vi "4_0_Signal operation in Time domain.vi"() -> ()   [LabVIEW 2009]
doc: "SIGNAL OPERATION allows users to generate and analyse signals and mathematical functions that operate on them."
uses:
  Instance          30 43Saved   4_0_Signal operation in Time domain .vi
  Instance          22 43Saved   4_0_Signal operation in Time domain .vi
  Instance          21 43Saved   4_0_Signal operation in Time domain .vi
  <vilib>/Analysis/2dsp.llb/1D Convolution (DBL).vi
  <vilib>/Analysis/2dsp.llb/1D Cross Correlation (DBL).vi
  <vilib>/Analysis/2dsp.llb/1D Auto Correlation (DBL).vi
  Instance          20 43Saved   4_0_Signal operation in Time domain .vi
  Instance          17 43Saved   4_0_Signal operation in Time domain .vi
  Instance          16 43Saved   4_0_Signal operation in Time domain .vi
  Instance          18 43Saved   4_0_Signal operation in Time domain .vi
  Instance          19 43Saved   4_0_Signal operation in Time domain .vi
  Instance          13 43Saved   4_0_Signal operation in Time domain .vi
  Instance          14 43Saved   4_0_Signal operation in Time domain .vi
  Instance          15 43Saved   4_0_Signal operation in Time domain .vi
  <vilib>/Analysis/NI_AALBase.lvlib
  <vilib>/Analysis/NI_AALPro.lvlib
panel:
  out "?":string="MULTIPLICATION\nPRESS \"SUPERIMPOSE\" TO SUPERIMPOSE SIGNALS"
  out "?":bool
  out "?":string="Time"
  out "?":string="Time"
  in  "?":bool
  in  "?":bool
  out "?":string="Sine wave.    Digitalized frequency = analog freq/sampling rate"
  out "?":string="Sine wave.    Digitalized frequency = analog freq/sampling rate"
  in  "alpha":dbl=0.95
  in  "c":dbl=1.0
  in  "Freq in cycles":dbl=1.0
  in  "Samp freq Fs":dbl=1000.0
  in  "Frequency Type":enum16{"Cycles", "Hz"}(ring)=enum."Hz"
  in  "Samp freq Fs":dbl=100.0
  in  "Freq in cycles":dbl=2.0
  in  "Frequency Type":enum16{"Cycles", "Hz"}(ring)=enum."Hz"
  in  "?":bool=TRUE
  out "OUTPUT ARRAY":dbl[](array[numeric])=[0.0, 0.036907341363112925, 0.11919898848967402, 0.1782102202687055, 0.14617624806978086, 1.640005609034487e-17, -0.2163781830748172, -0.40494016974649644, -0.45817497100356813, -0.3149510878717969, -6.238952084931405e-17, 0.3746684206317084, 0.6510429858044683, 0.6932903632838676, 0.452896320799659, 1.288077127857828e-16, -0.49628350270878235, -0.8334171783286888, -0.8605416643679448, -0.5465089063334351, -2.0189673055202066e-16, 0.5693188977302334, 0.9342106906791706, 0.9435571515973541, 0.5866253923638434, 2.653584817158272e-16, -0.5866253923638429, -0.9435571515973541, -0.934210690679171, -0.5693188977302339, -3.028450958280311e-16, 0.546508906333435, 0.860541664367945, 0.8334171783286893, 0.49628350270878313, 3.005513298334935e-16, -0.45289632079965925, -0.6932903632838684, -0.6510429858044695, -0.37466842063170946, -2.495580833972569e-16, 0.3149510878717977, 0.45817497100356985, 0.40494016974649855, 0.21637818307481868, 1.47600504813105e-16, -0.14617624806978222, -0.17821022026870806, -0.11919898848967671, -0.036907341363114674, -1.6077664410013713e-30, -0.03690734136311106, -0.11919898848967093, -0.17821022026870242, -0.146176248069779, -1.8040061699379165e-16, 0.2163781830748151, 0.40494016974649316, 0.45817497100356497, 0.3149510878717951, 3.743371250958822e-16, -0.3746684206317062, -0.6510429858044651, -0.6932903632838647, -0.45289632079965764, -5.5816675540505695e-16, 0.49628350270878047, 0.8334171783286862, 0.8605416643679429, 0.5465089063334344, 7.066385569320712e-16, -0.5693188977302323, -0.9342106906791695, -0.9435571515973538, -0.5866253923638437, -7.960754451474816e-16, 0.5866253923638426, 0.9435571515973542, 0.9342106906791715, 0.5693188977302346, 8.075869222080832e-16, -0.5465089063334346, -0.8605416643679449, -0.8334171783286893, -0.4962835027087831, -7.299103724527691e-16, 0.45289632079965814, 0.6932903632838667, 0.6510429858044675, 0.3746684206317082, 5.615056876438249e-16, -0.3149510878717952, -0.45817497100356575, -0.40494016974649394, -0.21637818307481566, -3.1160106571654887e-16, 0.14617624806977822, 0.17821022026870112, 0.11919898848966928, 0.03690734136310978]
  in  "Time Delay":dbl(slide) scale=0.0..1.0
  in  "?":T1(ring)=enum."BOTH SIGNALS"
  in  "?":bool
  in  "?":bool
  in  "stop":bool
  in  "?":T2(ring)=enum."MULTIPLICATION"
  in  "Delta t":dbl=0.1 format="%0.2f"
  in  "Width":i32=10
  in  "Wave Table":dbl[](array[numeric])=[1.0, 2.0, 3.0, 4.0]
  in  "Delta t":dbl=0.1 format="%0.2f"
  in  "Width":i32=1
  in  "Wave Table":dbl[](array[numeric])=[1.0, 2.0, 2.0, 3.0]
  in  "Delay":i32(knob)=15 scale=0.0..100.0
  in  "Signal 2 Pattern":T3(ring)
  in  "Delay":i32(knob) scale=0.0..100.0
  in  "Start":dbl format="%0.2f"
  in  "End":dbl=1.0 format="%0.2f"
  in  "Start":dbl format="%0.2f"
  in  "End":dbl=1.0 format="%0.2f"
  in  "Duty cycle (%)":dbl(knob)=50.0 step=1.0 scale=0.0..100.0
  in  "Duty cycle (%)":dbl=57.0 step=1.0
  in  "Phase in":dbl(knob) scale=0.0..180.0
  in  "Frequency in Hz":dbl(knob)=100.0 scale=0.0..5000.0 scale format="%#_6p"
  in  "Amplitude":dbl=1.0
  in  "Reset phase":bool=TRUE
  in  "Samples":i32=128
  in  "Phase in":dbl(knob) scale=0.0..180.0
  in  "Frequency in Hz":dbl(knob)=1.0 scale=0.0..5000.0 scale format="%#_6p"
  in  "Amplitude":dbl=1.0
  in  "Reset phase":bool=TRUE
  in  "Samples":i32=100
  in  "Signal 1 Pattern":T4(ring)
  out "Signal Operation (x,y)":dynamicdata(graph)=[{"t0"=timestamp(0 s since 1904-01-01), "dt"=1.0, "Y"=[0.0, 0.036907341363112925, 0.11919898848967402, 0.1782102202687055, 0.14617624806978086, 1.640005609034487e-17, -0.2163781830748172, -0.40494016974649644, -0.45817497100356813, -0.3149510878717969, -6.238952084931405e-17, 0.3746684206317084, 0.6510429858044683, 0.6932903632838676, 0.452896320799659, 1.288077127857828e-16, -0.49628350270878235, -0.8334171783286888, -0.8605416643679448, -0.5465089063334351, -2.0189673055202066e-16, 0.5693188977302334, 0.9342106906791706, 0.9435571515973541, 0.5866253923638434, 2.653584817158272e-16, -0.5866253923638429, -0.9435571515973541, -0.934210690679171, -0.5693188977302339, -3.028450958280311e-16, 0.546508906333435, 0.860541664367945, 0.8334171783286893, 0.49628350270878313, 3.005513298334935e-16, -0.45289632079965925, -0.6932903632838684, -0.6510429858044695, -0.37466842063170946, -2.495580833972569e-16, 0.3149510878717977, 0.45817497100356985, 0.40494016974649855, 0.21637818307481868, 1.47600504813105e-16, -0.14617624806978222, -0.17821022026870806, -0.11919898848967671, -0.036907341363114674, -1.6077664410013713e-30, -0.03690734136311106, -0.11919898848967093, -0.17821022026870242, -0.146176248069779, -1.8040061699379165e-16, 0.2163781830748151, 0.40494016974649316, 0.45817497100356497, 0.3149510878717951, 3.743371250958822e-16, -0.3746684206317062, -0.6510429858044651, -0.6932903632838647, -0.45289632079965764, -5.5816675540505695e-16, 0.49628350270878047, 0.8334171783286862, 0.8605416643679429, 0.5465089063334344, 7.066385569320712e-16, -0.5693188977302323, -0.9342106906791695, -0.9435571515973538, -0.5866253923638437, -7.960754451474816e-16, 0.5866253923638426, 0.9435571515973542, 0.9342106906791715, 0.5693188977302346, 8.075869222080832e-16, -0.5465089063334346, -0.8605416643679449, -0.8334171783286893, -0.4962835027087831, -7.299103724527691e-16, 0.45289632079965814, 0.6932903632838667, 0.6510429858044675, 0.3746684206317082, 5.615056876438249e-16, -0.3149510878717952, -0.45817497100356575, -0.40494016974649394, -0.21637818307481566, -3.1160106571654887e-16, 0.14617624806977822, 0.17821022026870112, 0.11919898848966928, 0.03690734136310978]}]
  out "Sequence y[n]":cluster{dbl, dbl, "bernoulli noise":dbl[]}(graph)={0.0, 0.001, "bernoulli noise"=[0.0, 0.5877852522924731, 0.9510565162951535, 0.9510565162951535, 0.5877852522924731, 5.307169634316544e-17, -0.587785252292473, -0.9510565162951535, -0.9510565162951536, -0.5877852522924732, -1.0614339268633088e-16, 0.587785252292473, 0.9510565162951535, 0.9510565162951536, 0.5877852522924732, 1.5921508902949633e-16, -0.587785252292473, -0.9510565162951535, -0.9510565162951536, -0.5877852522924732, -2.1228678537266177e-16, 0.5877852522924729, 0.9510565162951535, 0.9510565162951536, 0.5877852522924734, 2.653584817158272e-16, -0.5877852522924729, -0.9510565162951535, -0.9510565162951536, -0.5877852522924734, -3.1843017805899265e-16, 0.5877852522924729, 0.9510565162951534, 0.9510565162951536, 0.5877852522924735, 3.715018744021581e-16, -0.5877852522924728, -0.9510565162951534, -0.9510565162951536, -0.5877852522924735, -4.2457357074532354e-16, 0.5877852522924728, 0.9510565162951534, 0.9510565162951538, 0.5877852522924735, 4.77645267088489e-16, -0.5877852522924727, -0.9510565162951534, -0.9510565162951538, -0.5877852522924736, -5.307169634316544e-16, 0.5877852522924727, 0.9510565162951534, 0.9510565162951538, 0.5877852522924736, 5.837886597748199e-16, -0.5877852522924727, -0.9510565162951534, -0.9510565162951538, -0.5877852522924736, -6.368603561179853e-16, 0.5877852522924726, 0.9510565162951534, 0.9510565162951538, 0.5877852522924737, 6.899320524611507e-16, -0.5877852522924726, -0.9510565162951533, -0.9510565162951538, -0.5877852522924737, -7.430037488043162e-16, 0.5877852522924725, 0.9510565162951533, 0.9510565162951539, 0.5877852522924738, 7.960754451474816e-16, -0.5877852522924725, -0.9510565162951533, -0.9510565162951539, -0.5877852522924738, -8.491471414906471e-16, 0.5877852522924725, 0.9510565162951533, 0.9510565162951539, 0.5877852522924738, 9.022188378338125e-16, -0.5877852522924724, -0.9510565162951533, -0.9510565162951539, -0.5877852522924739, -9.55290534176978e-16, 0.5877852522924724, 0.9510565162951533, 0.9510565162951539, 0.5877852522924739, 1.0083622305201434e-15, -0.5877852522924724, -0.9510565162951533, -0.9510565162951539, -0.587785252292474, -1.0614339268633088e-15, 0.5877852522924722, 0.9510565162951532, 0.9510565162951539, 0.587785252292474, 1.1145056232064743e-15, -0.5877852522924722, -0.9510565162951532, -0.951056516295154, -0.587785252292474, -1.1675773195496397e-15, 0.5877852522924721, 0.9510565162951532, 0.951056516295154, 0.5877852522924741, 1.2206490158928052e-15, -0.5877852522924721, -0.9510565162951532, -0.951056516295154, -0.5877852522924741, -1.2737207122359706e-15, 0.5877852522924721, 0.9510565162951532, 0.951056516295154, 0.5877852522924742, 1.326792408579136e-15, -0.587785252292472, -0.9510565162951532]}
  out "Sequence x[n]":cluster{dbl, dbl, "Waveform Graph":dbl[]}(graph)={0.0, 0.01, "Waveform Graph"=[0.0, 0.06279051952931337, 0.12533323356430426, 0.18738131458572463, 0.2486898871648548, 0.3090169943749474, 0.368124552684678, 0.42577929156507266, 0.4817536741017153, 0.5358267949789967, 0.5877852522924732, 0.6374239897486899, 0.6845471059286888, 0.7289686274214117, 0.7705132427757894, 0.8090169943749476, 0.8443279255020152, 0.8763066800438637, 0.9048270524660196, 0.9297764858882515, 0.9510565162951535, 0.9685831611286311, 0.9822872507286886, 0.9921147013144778, 0.9980267284282716, 1.0, 0.9980267284282716, 0.9921147013144779, 0.9822872507286888, 0.9685831611286313, 0.9510565162951539, 0.9297764858882518, 0.90482705246602, 0.8763066800438643, 0.8443279255020159, 0.8090169943749483, 0.7705132427757903, 0.7289686274214127, 0.6845471059286901, 0.6374239897486912, 0.5877852522924748, 0.5358267949789984, 0.4817536741017172, 0.42577929156507477, 0.3681245526846802, 0.30901699437494984, 0.24868988716485732, 0.18738131458572732, 0.12533323356430706, 0.0627905195293163, 3.0294235002503722e-15, -0.06279051952931025, -0.12533323356430104, -0.18738131458572135, -0.24868988716485146, -0.30901699437494407, -0.3681245526846746, -0.4257792915650693, -0.48175367410171194, -0.5358267949789933, -0.5877852522924699, -0.6374239897486865, -0.6845471059286856, -0.7289686274214086, -0.7705132427757864, -0.8090169943749448, -0.8443279255020126, -0.8763066800438613, -0.9048270524660175, -0.9297764858882496, -0.951056516295152, -0.9685831611286299, -0.9822872507286877, -0.9921147013144772, -0.9980267284282713, -1.0, -0.9980267284282718, -0.9921147013144782, -0.9822872507286892, -0.9685831611286317, -0.9510565162951542, -0.929776485888252, -0.90482705246602, -0.876306680043864, -0.8443279255020153, -0.8090169943749475, -0.770513242775789, -0.728968627421411, -0.6845471059286878, -0.6374239897486885, -0.5877852522924716, -0.5358267949789947, -0.48175367410171294, -0.4257792915650699, -0.36812455268467476, -0.30901699437494373, -0.24868988716485066, -0.18738131458572005, -0.12533323356429923, -0.06279051952930793]}
  # "Program Developed by Indranil Sinharoy"
  # "Message Box"
  # "Signal/Sequence x(n)"
  # "Real Exponential"
  # "Impulse/Pulse/Sinc\n/Step"
  # "Pulse"
  # "Sinc"
  # "Ramp char."
  # "Square Wave char."
  # "Arbitrary Waveform (Point by Point)"
  # "SIGNAL OPERATION"
  # "Signal/Sequence y(n)"
  # "Pulse"
  # "Sinc"
  # "Square Wave char."
  # "Impulse/Pulse/Sinc\n/Step"
  # "Ramp char."
  # "Arbitrary Waveform (Point by Point)"
  # "y[n]"
  # "x[n]"
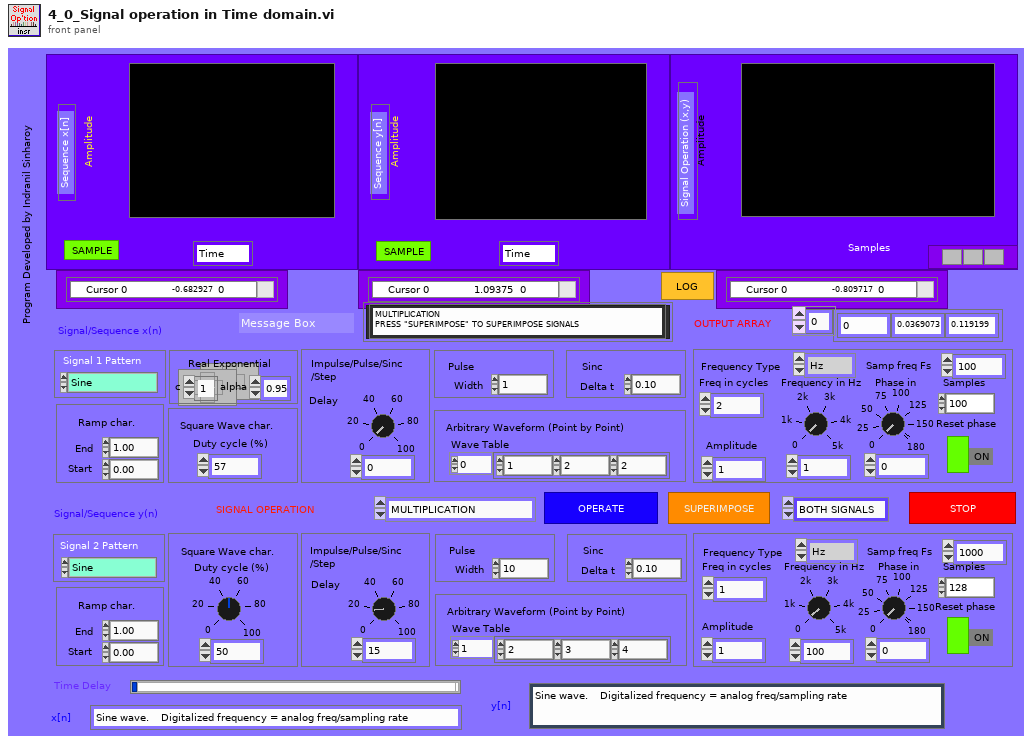
[diagram p1: front panel]
types:
  T1 = enum16{"NO SIGNAL", "SIGNAL x[n]", "SIGNAL y[n]", "BOTH SIGNALS"}
  T2 = enum16{"CONVOLUTION", "ADDITION", "MULTIPLICATION", "CROSS CORRELATION", "AUTO CORRELATION", "BACKWARD DIFFERENCE", "ACCUMULATOR FUNCTION"}
  T3 = enum16{"Sine", "Square", "Ramp", "Triangular", "Sawtooth", "Pulse wave", "Impulse", "Step", "Sinc Pattern", "Arbitrary wave", "Unif. white noise", "Gaussian white noise", "Periodic rand noise", "Gamma noise", "Poisson noise", "Binomial noise", "Bernoulli noise"}
  T4 = enum16{"Sine", "Square", "Ramp", "Triangular", "Sawtooth", "Pulse wave", "Impulse", "Step", "Sinc Pattern", "Arbitrary wave", "Real Exponential", "Chirp Pattern"}
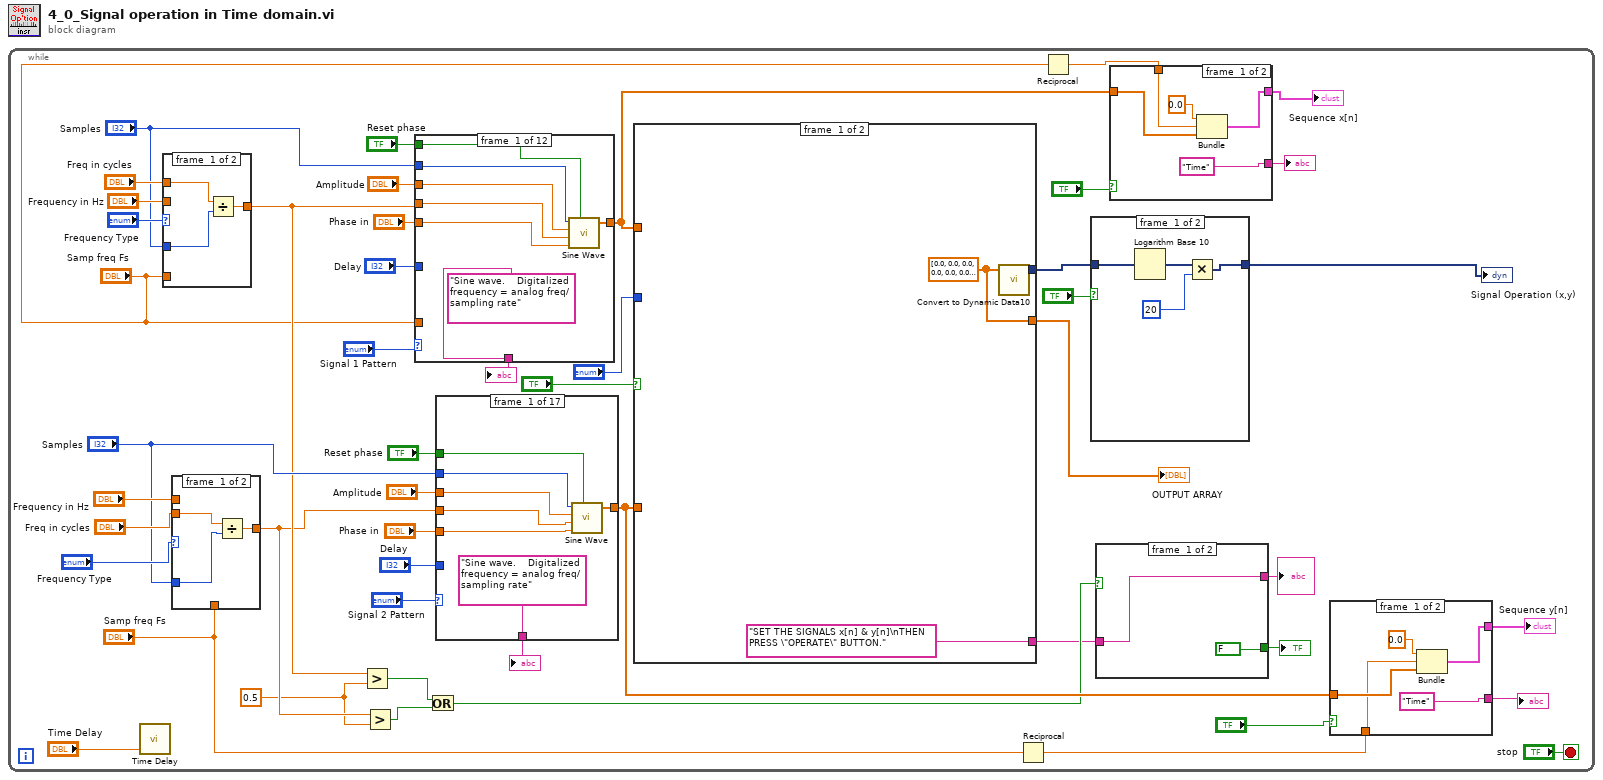
[diagram p0: block diagram]
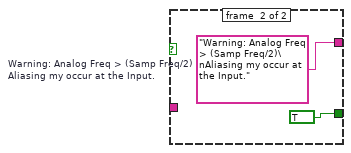
[diagram p2: hidden frame]
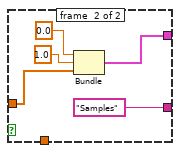
[diagram p3: hidden frame]
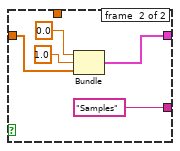
[diagram p4: hidden frame]
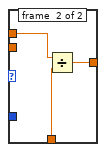
[diagram p5: hidden frame]
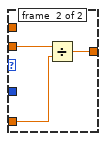
[diagram p6: hidden frame]
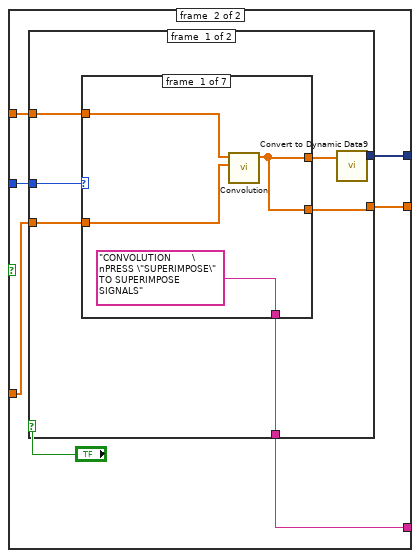
[diagram p8: hidden frame]
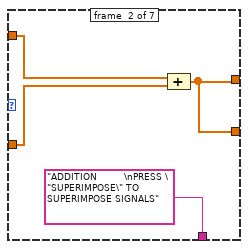
[diagram p9: hidden frame]
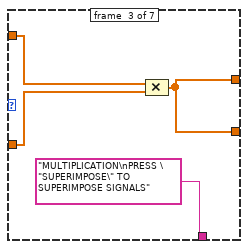
[diagram p10: hidden frame]
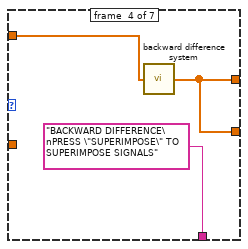
[diagram p11: hidden frame]
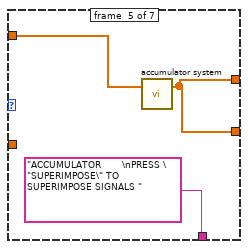
[diagram p12: hidden frame]
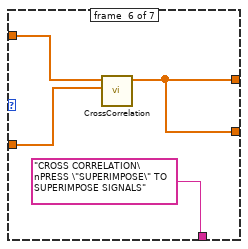
[diagram p13: hidden frame]
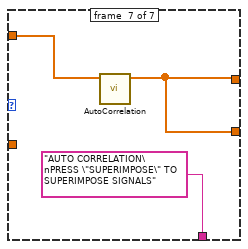
[diagram p14: hidden frame]
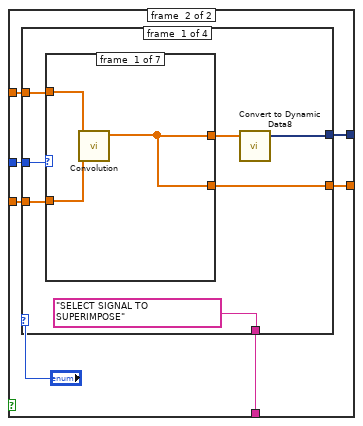
[diagram p15: hidden frame]
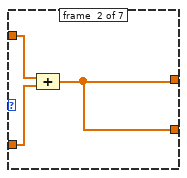
[diagram p16: hidden frame]
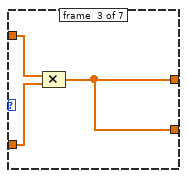
[diagram p17: hidden frame]
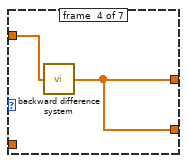
[diagram p18: hidden frame]
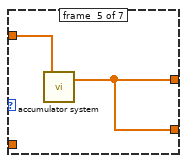
[diagram p19: hidden frame]
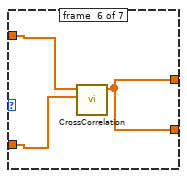
[diagram p20: hidden frame]
diagram:
  n1 = while {
    stop <- "stop" stop-if-true
    w6 = 0.5
    n2 = call "Time Delay"("Delay Time (s)"="Time Delay") -> ()  [unwired: 10 in, 1 out]
    n3 = case shown="\"Cycles\", Default" "Frequency Type" {
      tunnel: "Frequency in Hz" -> [_ w85]
      tunnel: "Freq in cycles" -> [w81 _]
      tunnel: "Samp freq Fs" -> [_ w84]
      tunnel: [w82 w83] -> w9
      tunnel: "Samples" -> [w80 _]
      frame #0 {
        n4 = Divide(x=w81, y=w80) -> (x/y=w82:dbl)
      }
      frame #1 {
        n5 = Divide(x=w85, y=w84) -> (x/y=w83:dbl)
      }
    }
    n6 = case shown="\"Cycles\", Default" "Frequency Type" {
      tunnel: [w76 w79] -> w7
      tunnel: "Frequency in Hz" -> [_ w78]
      tunnel: "Freq in cycles" -> [w75 _]
      tunnel: "Samp freq Fs" -> [_ w77]
      tunnel: "Samples" -> [w74 _]
      frame #0 {
        n7 = Divide(x=w75, y=w74) -> (x/y=w76:dbl)
      }
      frame #1 {
        n8 = Divide(x=w78, y=w77) -> (x/y=w79:dbl)
      }
    }
    n9 = Greater?(x=w9, y=w6) -> (0:w11:bool)
    n10 = Greater?(x=w7, y=w6) -> (0:w10:bool)
    n11 = case shown="\"Chirp Pattern\"" "Signal 1 Pattern" {
      tunnel: "Samples" -> [w377 w384 w390 w396 w403 w409 _ w417 w423 w427 w432 w439]
      tunnel: "Reset phase" -> [w376 w385 _ w397 w404 _ _ _ _ _ _ _]
      tunnel: "Amplitude" -> [w375 w383 _ w395 w402 w408 _ w416 w422 _ _ w438]
      tunnel: w9 -> [w374 w382 _ w394 w401 _ _ _ _ _ _ w434]
      tunnel: "Phase in" -> [w373 w381 _ w393 w400 _ _ _ _ _ _ _]
      tunnel: [w372 w380 w389 w392 w399 w407 "Wave Table" w414 w420 w425 w429 w440] -> w36
      tunnel: "Delay" -> [_ _ _ _ _ w406 _ w415 w421 w426 _ w437]
      tunnel: ["Sine wave.    Digitalized frequency = analog freq/sampling rate" "Square wave.    Digitalized frequency = analog freq/sampling rate" " Ramp.    Digitalized frequency = analog freq/sampling rate" "Triangular wave.    Digitalized frequency = analog freq/sampling rate" "Sawtooth wave.    Digitalized frequency = analog freq/sampling rate" "Impulse Function. Vary the delay to generate impulse at delayed instant." "Create arbitrary sequence by specifying values in the wave table" "Pulse. Vary the delay to generate Pulse at delayed instant." "Sinc pattern. Vary the delay to generate sinc at delayed instant." "Step function. Vary the delay to generate step at delayed instant." w428 "Chirp pattern. Vary delay knob to set f1 & freq knob to set f2."] -> w8
      tunnel: "Samp freq Fs" -> [_ _ _ _ _ _ _ _ _ _ _ w436]
      frame #0 {
        n12 = call <vilib>:"Sine Wave.vi"("samples"=w377, "amplitude"=w375, "frequency"=w374, "phase in"=w373, "reset phase"=w376) -> ("sine wave"=w372:dbl[])  [unwired: 2 out]
      }
      frame #1 {
        n13 = call <vilib>:"Square Wave.vi"("samples"=w384, "reset phase"=w385, "amplitude"=w383, "frequency"=w382, "duty cycle (%)"="Duty cycle (%)", "phase in"=w381) -> ("square wave"=w380:dbl[])  [unwired: 2 out]
      }
      frame #2 {
        n14 = call <vilib>:"Ramp Pattern.vi"("start"="Start", "end"="End", "samples"=w390) -> ("Ramp Pattern"=w389:dbl[])  [unwired: 7 in, 1 out]
      }
      frame #3 {
        n15 = call <vilib>:"Triangle Wave.vi"("samples"=w396, "amplitude"=w395, "frequency"=w394, "phase in"=w393, "reset phase"=w397) -> ("triangle wave"=w392:dbl[])  [unwired: 2 out]
      }
      frame #4 {
        n16 = call <vilib>:"Sawtooth Wave.vi"("samples"=w403, "amplitude"=w402, "frequency"=w401, "phase in"=w400, "reset phase"=w404) -> ("sawtooth wave"=w399:dbl[])  [unwired: 2 out]
      }
      frame #5 {
        n17 = call <vilib>:"Impulse Pattern.vi"("delay"=w406, "amplitude"=w408, "samples"=w409) -> ("Impulse Pattern"=w407:dbl[])  [unwired: 1 out]
      }
      frame #6 {
      }
      frame #7 {
        n18 = call <vilib>:"Pulse Pattern.vi"("width"="Width", "delay"=w415, "amplitude"=w416, "samples"=w417) -> ("Pulse Pattern"=w414:dbl[])  [unwired: 1 out]
      }
      frame #8 {
        n19 = call <vilib>:"Sinc Pattern.vi"("delta t"="Delta t", "delay"=w421, "amplitude"=w422, "samples"=w423) -> ("Sinc Pattern"=w420:dbl[])  [unwired: 1 out]
      }
      frame #9 {
        n20 = call "stepinput_numarray.vi"("Step Delay"=w426, "Samples"=w427) -> ("OUTPUT ARRAY"=w425:dbl[])
      }
      frame #10 {
        w428 = "Real exponential sequence  x[n] = C*alpha^n"  # Real exponential sequence  x[n] = C*alpha^n
        n21 = call "C alpha to the power n.vi"("alpha"="alpha", "c"="c", "n"=w432) -> ("Waveform Graph"=w429:dbl[])
      }
      frame #11 {
        n22 = Divide(x=w437, y=w436) -> (x/y=w435:dbl)
        n23 = call <vilib>:"Chirp Pattern.vi"("f2"=w434, "f1"=w435, "amplitude"=w438, "samples"=w439) -> ("Chirp Pattern"=w440:dbl[])  [unwired: 1 out]
      }
    }
    "?" <- w8
    n24 = Or(x=w11, y=w10) -> (x .or. y?=w5:bool)
    n25 = case shown="\"Sinc Pattern\"" "Signal 2 Pattern" {
      tunnel: "Reset phase" -> [w284 w287 _ w304 w310 _ _ _ _ _ _ _ _ _ _ _ _]
      tunnel: "Samples" -> [w283 w288 w297 w303 w309 w317 w320 w328 _ w334 w339 w343 w348 w353 w358 w364 w369]
      tunnel: "Amplitude" -> [w282 w289 _ w302 w308 w316 w321 w327 _ _ w338 _ w347 _ _ _ _]
      tunnel: "Phase in" -> [w281 w290 _ w301 w307 _ _ _ _ _ _ _ _ _ _ _ _]
      tunnel: [w280 w291 w296 w300 w311 w314 w319 w325 "Wave Table" w333 w337 w344 w349 w354 w359 w365 w370] -> w15
      tunnel: "Delay" -> [_ _ _ _ _ w315 w322 w326 _ w332 _ _ _ _ _ _ _]
      tunnel: w7 -> [w279 w286 _ w299 w306 _ _ _ _ _ _ _ _ _ _ _ _]
      tunnel: ["Sine wave.    Digitalized frequency = analog freq/sampling rate" "Square wave.    Digitalized frequency = analog freq/sampling rate" " Ramp.    Digitalized frequency = analog freq/sampling rate" "Triangular wave.    Digitalized frequency = analog freq/sampling rate" "Sawtooth wave.    Digitalized frequency = analog freq/sampling rate" "Pulse. Vary the delay to generate Pulse at delayed instant." "Impulse Function. Vary the delay to generate impulse at delayed instant." "Sinc pattern. Vary the delay to generate sinc at delayed instant." "Create arbitrary sequence by specifying values in the wave table" "Step function. Vary the delay to generate step at delayed instant." "Uniform White Noise. Seed has been set to -1. The amplitude & no. of samples can be varied." "Gaussian White Noise. Seed has been set to -1, standard deviation to 1. The no. of samples can be varied." "Periodic Random Noise. Seed has been set to -1. The amplitude & no. of samples can be varied." "Gamma Noise. Seed has been set to -1, order to 1. The no. of samples can be varied." "Poisson Noise. Seed has been set to -1, mean to 1. The no. of samples can be varied." "Binomial Noise. Seed has been set to -1, trials to 1 and trial probability to 0.5 . The no. of samples can be varied." "Bernoulli Noise. Seed has been set to -1 and ones probability to 0.5 . The no. of samples can be varied."] -> w23
      frame #0 {
        n26 = call <vilib>:"Sine Wave.vi"("samples"=w283, "amplitude"=w282, "frequency"=w279, "phase in"=w281, "reset phase"=w284) -> ("sine wave"=w280:dbl[])  [unwired: 2 out]
      }
      frame #1 {
        n27 = call <vilib>:"Square Wave.vi"("samples"=w288, "reset phase"=w287, "amplitude"=w289, "frequency"=w286, "duty cycle (%)"="Duty cycle (%)", "phase in"=w290) -> ("square wave"=w291:dbl[])  [unwired: 2 out]
      }
      frame #2 {
        n28 = call <vilib>:"Ramp Pattern.vi"("start"="Start", "end"="End", "samples"=w297) -> ("Ramp Pattern"=w296:dbl[])  [unwired: 7 in, 1 out]
      }
      frame #3 {
        n29 = call <vilib>:"Triangle Wave.vi"("samples"=w303, "amplitude"=w302, "frequency"=w299, "phase in"=w301, "reset phase"=w304) -> ("triangle wave"=w300:dbl[])  [unwired: 2 out]
      }
      frame #4 {
        n30 = call <vilib>:"Sawtooth Wave.vi"("samples"=w309, "amplitude"=w308, "frequency"=w306, "phase in"=w307, "reset phase"=w310) -> ("sawtooth wave"=w311:dbl[])  [unwired: 2 out]
      }
      frame #5 {
        n31 = call <vilib>:"Pulse Pattern.vi"("width"="Width", "delay"=w315, "amplitude"=w316, "samples"=w317) -> ("Pulse Pattern"=w314:dbl[])  [unwired: 1 out]
      }
      frame #6 {
        n32 = call <vilib>:"Impulse Pattern.vi"("delay"=w322, "amplitude"=w321, "samples"=w320) -> ("Impulse Pattern"=w319:dbl[])  [unwired: 1 out]
      }
      frame #7 {
        n33 = call <vilib>:"Sinc Pattern.vi"("delta t"="Delta t", "delay"=w326, "amplitude"=w327, "samples"=w328) -> ("Sinc Pattern"=w325:dbl[])  [unwired: 1 out]
      }
      frame #8 {
      }
      frame #9 {
        n34 = call "stepinput_numarray.vi"("Step Delay"=w332, "Samples"=w334) -> ("OUTPUT ARRAY"=w333:dbl[])
      }
      frame #10 {
        n35 = call <vilib>:"Uniform White Noise (obs 90).vi"("seed"=-1, "amplitude"=w338, "samples"=w339) -> ("uniform white noise"=w337:dbl[])  [unwired: 1 out]
      }
      frame #11 {
        n36 = call <vilib>:"Gaussian White Noise (obs 90).vi"("seed"=-1, "standard deviation"=1.0000000000000002, "samples"=w343) -> ("Gaussian noise pattern"=w344:dbl[])  [unwired: 1 out]
      }
      frame #12 {
        n37 = call <vilib>:"Periodic Random Noise.vi"("seed"=-1, "spectral amplitude"=w347, "samples"=w348) -> ("periodic random noise"=w349:dbl[])  [unwired: 1 out]
      }
      frame #13 {
        n38 = call <vilib>:"Gamma Noise (obs 90).vi"("seed"=-1, "order"=1, "samples"=w353) -> ("gamma noise"=w354:dbl[])  [unwired: 1 out]
      }
      frame #14 {
        n39 = call <vilib>:"Poisson Noise (obs 90).vi"("seed"=-1, "mean"=1.0, "samples"=w358) -> ("poisson noise"=w359:dbl[])  [unwired: 1 out]
      }
      frame #15 {
        n40 = call <vilib>:"Binomial Noise (obs 90).vi"("seed"=-1, "trial probability"=0.5, "trials"=1, "samples"=w364) -> ("binomial noise"=w365:u32[])  [unwired: 1 out]
      }
      frame #16 {
        n41 = call <vilib>:"Bernoulli Noise (obs 90).vi"("seed"=-1, "ones probability"=0.5, "samples"=w369) -> ("bernoulli noise"=w370:u8[])  [unwired: 1 out]
      }
    }
    "?" <- w23
    n42 = case shown="True" "?" {
      tunnel: "?" -> [_ w100]
      tunnel: w36 -> [_ w99]
      tunnel: w15 -> [_ w98]
      tunnel: [w93 w96] -> w33
      tunnel: ["SET THE SIGNALS x[n] & y[n]\nTHEN PRESS \"OPERATE\" BUTTON." w95] -> w4
      tunnel: [w91 w94] -> w34
      frame #0 {
        w91 = dbl[] [0.0, 0.0, 0.0, 0.0, 0.0, 0.0, 0.0, 0.0, 0.0, 0.0, 0.0, 0.0, 0.0, 0.0, 0.0, 0.0, 0.0, 0.0, 0.0, 0.0, 0.0, 0.0, 0.0, 0.0, 0.0, 0.0, 0.0, 0.0, 0.0, 0.0, 0.0, 0.0, 0.0, 0.0, 0.0, 0.0, 0.0, 0.0, 0.0, 0.0, 0.0, 0.0, 0.0, 0.0, 0.0, 0.0, 0.0, 0.0, 0.0, 0.0, 0.0, 0.0, 0.0, 0.0, 0.0, 0.0, 0.0, 0.0, 0.0, 0.0, 0.0, 0.0, 0.0, 0.0, 0.0, 0.0, 0.0, 0.0, 0.0, 0.0, 0.0, 0.0, 0.0, 0.0, 0.0, 0.0, 0.0, 0.0, 0.0, 0.0, 0.0, 0.0, 0.0, 0.0, 0.0, 0.0, 0.0, 0.0, 0.0, 0.0, 0.0, 0.0, 0.0, 0.0, 0.0, 0.0, 0.0, 0.0, 0.0, 0.0, 0.0] ("X * Y")
        n43 = call "Convert to Dynamic Data10"("Array"=w91) -> ("Dynamic Data Type"=w93:dynamicdata)  [unwired: 3 in]
      }
      frame #1 {
        n44 = case shown="True" "?" {
          tunnel: w100 -> [w105 w139]
          tunnel: w99 -> [w107 w138]
          tunnel: w98 -> [w106 w137]
          tunnel: [w103 w135] -> w96
          tunnel: [w102 w134] -> w95
          tunnel: [w101 w133] -> w94
          frame #0 {
            n45 = case shown="\"MULTIPLICATION\"" w105 {
              tunnel: w107 -> [w111 w115 w119 w122 w125 w128 w131]
              tunnel: w106 -> [w110 w114 w118 _ _ w126 _]
              tunnel: [w108 w112 w116 w120 w123 w127 w130] -> w104
              tunnel: ["CONVOLUTION       \nPRESS \"SUPERIMPOSE\" TO SUPERIMPOSE SIGNALS" "ADDITION         \nPRESS \"SUPERIMPOSE\" TO SUPERIMPOSE SIGNALS" "MULTIPLICATION\nPRESS \"SUPERIMPOSE\" TO SUPERIMPOSE SIGNALS" "BACKWARD DIFFERENCE\nPRESS \"SUPERIMPOSE\" TO SUPERIMPOSE SIGNALS" "ACCUMULATOR       \nPRESS \"SUPERIMPOSE\" TO SUPERIMPOSE SIGNALS " "CROSS CORRELATION\nPRESS \"SUPERIMPOSE\" TO SUPERIMPOSE SIGNALS" "AUTO CORRELATION\nPRESS \"SUPERIMPOSE\" TO SUPERIMPOSE SIGNALS"] -> w102
              tunnel: [w108 w112 w116 w120 w123 w127 w130] -> w101
              frame #0 {
                n46 = call-poly <vilib>:"Convolution.vi"("Y"=w110, "X"=w111) -> ("X * Y"=w108:dbl[])  [unwired: 8 in, 1 out]
              }
              frame #1 {
                n47 = Compound Arithmetic op=ADD(w115, w114) -> (w112:dbl[])
              }
              frame #2 {
                n48 = Compound Arithmetic op=MULTIPLY(w119, w118) -> (w116:dbl[])
              }
              frame #3 {
                n49 = call "backward difference system.vi"("Input sequence x[n]"=w122) -> ("B[n] = x[n] - x[n-1]"=w120:dbl[])
              }
              frame #4 {
                n50 = call "accumulator system.vi"("Sequence x[n]"=w125) -> ("Accumulated sequence A[n] = Sum(k: k ( -infinity to n) x[k]"=w123:dbl[])  [unwired: 2 out]
              }
              frame #5 {
                n51 = call-poly <vilib>:"CrossCorrelation.vi"("Y"=w126, "X"=w128) -> ("Rxy"=w127:dbl[])  [unwired: 8 in, 1 out]
              }
              frame #6 {
                n52 = call-poly <vilib>:"AutoCorrelation.vi"("X"=w131) -> ("Rxx"=w130:dbl[])  [unwired: 9 in, 1 out]
              }
            }
            n53 = call "Convert to Dynamic Data9"("Array"=w104) -> ("Dynamic Data Type"=w103:dynamicdata)  [unwired: 3 in]
          }
          frame #1 {
            n54 = case shown="\"SIGNAL x[n]\"" "?" {
              tunnel: w139 -> [w144 w174 w207 w247]
              tunnel: w138 -> [w146 w173 w209 w249]
              tunnel: w137 -> [w145 w172 w208 w248]
              tunnel: [w142 w167 w202 w240] -> w135
              tunnel: ["SELECT SIGNAL TO SUPERIMPOSE" w166 w201 w239] -> w134
              tunnel: [w140 w165 w200 w238] -> w133
              frame #0 {
                n55 = case shown="\"MULTIPLICATION\"" w144 {
                  tunnel: w146 -> [w149 w152 w155 w157 w159 w161 w163]
                  tunnel: w145 -> [w148 w151 w154 _ _ w160 _]
                  tunnel: [w147 w150 w153 w156 w158 w162 w164] -> w143
                  tunnel: [w147 w150 w153 w156 w158 w162 w164] -> w140
                  frame #0 {
                    n56 = call-poly <vilib>:"Convolution.vi"("Y"=w148, "X"=w149) -> ("X * Y"=w147:dbl[])  [unwired: 8 in, 1 out]
                  }
                  frame #1 {
                    n57 = Compound Arithmetic op=ADD(w152, w151) -> (w150:dbl[])
                  }
                  frame #2 {
                    n58 = Compound Arithmetic op=MULTIPLY(w155, w154) -> (w153:dbl[])
                  }
                  frame #3 {
                    n59 = call "backward difference system.vi"("Input sequence x[n]"=w157) -> ("B[n] = x[n] - x[n-1]"=w156:dbl[])
                  }
                  frame #4 {
                    n60 = call "accumulator system.vi"("Sequence x[n]"=w159) -> ("Accumulated sequence A[n] = Sum(k: k ( -infinity to n) x[k]"=w158:dbl[])  [unwired: 2 out]
                  }
                  frame #5 {
                    n61 = call-poly <vilib>:"CrossCorrelation.vi"("Y"=w160, "X"=w161) -> ("Rxy"=w162:dbl[])  [unwired: 8 in, 1 out]
                  }
                  frame #6 {
                    n62 = call-poly <vilib>:"AutoCorrelation.vi"("X"=w163) -> ("Rxx"=w164:dbl[])  [unwired: 9 in, 1 out]
                  }
                }
                n63 = call "Convert to Dynamic Data8"("Array"=w143) -> ("Dynamic Data Type"=w142:dynamicdata)  [unwired: 3 in]
              }
              frame #1 {
                n64 = case shown="\"MULTIPLICATION\"" w174 {
                  tunnel: w173 -> [w177 w181 w185 w189 w192 w194 w199]
                  tunnel: w172 -> [w178 w182 w186 _ _ w195 _]
                  tunnel: [w175 w179 w183 w187 w190 w196 w198] -> w169
                  tunnel: [w177 w181 w185 w189 w192 w194 w199] -> w171
                  tunnel: ["CONVOLUTION        \n" "ADDITIION        \n" "MULTIPLICATION        \n" "BACKWARD DIFFERENCE        \n" "ACCUMULATOR FUNCTION        \n" "CROSS CORRELATION" "AUTO CORRELATION"] -> w166
                  tunnel: [w175 w179 w183 w187 w190 w196 w198] -> w165
                  frame #0 {
                    n65 = call-poly <vilib>:"Convolution.vi"("Y"=w178, "X"=w177) -> ("X * Y"=w175:dbl[])  [unwired: 8 in, 1 out]
                  }
                  frame #1 {
                    n66 = Compound Arithmetic op=ADD(w181, w182) -> (w179:dbl[])
                  }
                  frame #2 {
                    n67 = Compound Arithmetic op=MULTIPLY(w185, w186) -> (w183:dbl[])
                  }
                  frame #3 {
                    n68 = call "backward difference system.vi"("Input sequence x[n]"=w189) -> ("B[n] = x[n] - x[n-1]"=w187:dbl[])
                  }
                  frame #4 {
                    n69 = call "accumulator system.vi"("Sequence x[n]"=w192) -> ("Accumulated sequence A[n] = Sum(k: k ( -infinity to n) x[k]"=w190:dbl[])  [unwired: 2 out]
                  }
                  frame #5 {
                    n70 = call-poly <vilib>:"CrossCorrelation.vi"("Y"=w195, "X"=w194) -> ("Rxy"=w196:dbl[])  [unwired: 8 in, 1 out]
                  }
                  frame #6 {
                    n71 = call-poly <vilib>:"AutoCorrelation.vi"("X"=w199) -> ("Rxx"=w198:dbl[])  [unwired: 9 in, 1 out]
                  }
                }
                n72 = call "Convert to Dynamic Data4"("Array"=w171) -> ("Dynamic Data Type"=w170:dynamicdata)  [unwired: 3 in]
                n73 = call "Convert to Dynamic Data5"("Array"=w169) -> ("Dynamic Data Type"=w168:dynamicdata)  [unwired: 3 in]
                n74 = Merge Signals(w170, w168) -> (w167:dynamicdata)
              }
              frame #2 {
                n75 = case shown="\"MULTIPLICATION\"" w207 {
                  tunnel: w209 -> [w213 w217 w221 w225 w229 w232 w237]
                  tunnel: w208 -> [w212 w216 w220 _ _ w231 w235]
                  tunnel: [w210 w214 w218 w222 w226 w233 w236] -> w203
                  tunnel: [w212 w216 w220 dbl[] [0.0, 0.0, 0.0, 0.0, 0.0, 0.0, 0.0, 0.0, 0.0, 0.0, 0.0, 0.0, 0.0, 0.0, 0.0, 0.0, 0.0, 0.0, 0.0, 0.0, 0.0, 0.0, 0.0, 0.0, 0.0, 0.0, 0.0, 0.0, 0.0, 0.0, 0.0, 0.0, 0.0, 0.0, 0.0, 0.0, 0.0, 0.0, 0.0, 0.0, 0.0, 0.0, 0.0, 0.0, 0.0, 0.0, 0.0, 0.0, 0.0, 0.0, 0.0, 0.0, 0.0, 0.0, 0.0, 0.0, 0.0, 0.0, 0.0, 0.0, 0.0, 0.0, 0.0, 0.0, 0.0, 0.0, 0.0, 0.0, 0.0, 0.0, 0.0, 0.0, 0.0, 0.0, 0.0, 0.0, 0.0, 0.0, 0.0, 0.0, 0.0, 0.0, 0.0, 0.0, 0.0, 0.0, 0.0, 0.0, 0.0, 0.0, 0.0, 0.0, 0.0, 0.0, 0.0, 0.0, 0.0, 0.0, 0.0, 0.0, 0.0] dbl[] [0.0, 0.0, 0.0, 0.0, 0.0, 0.0, 0.0, 0.0, 0.0, 0.0, 0.0, 0.0, 0.0, 0.0, 0.0, 0.0, 0.0, 0.0, 0.0, 0.0, 0.0, 0.0, 0.0, 0.0, 0.0, 0.0, 0.0, 0.0, 0.0, 0.0, 0.0, 0.0, 0.0, 0.0, 0.0, 0.0, 0.0, 0.0, 0.0, 0.0, 0.0, 0.0, 0.0, 0.0, 0.0, 0.0, 0.0, 0.0, 0.0, 0.0, 0.0, 0.0, 0.0, 0.0, 0.0, 0.0, 0.0, 0.0, 0.0, 0.0, 0.0, 0.0, 0.0, 0.0, 0.0, 0.0, 0.0, 0.0, 0.0, 0.0, 0.0, 0.0, 0.0, 0.0, 0.0, 0.0, 0.0, 0.0, 0.0, 0.0, 0.0, 0.0, 0.0, 0.0, 0.0, 0.0, 0.0, 0.0, 0.0, 0.0, 0.0, 0.0, 0.0, 0.0, 0.0, 0.0, 0.0, 0.0, 0.0, 0.0, 0.0] w231 w235] -> w204
                  tunnel: ["CONVOLUTION        \n" "ADDITION            \n" "MULTIPLICATION        \n" "BACKWARD DIFFERENCE  \n" "ACCUMULATOR         \n" "CROSS CORRELATION" "AUTO CORRELATION"] -> w201
                  tunnel: [w210 w214 w218 w222 w226 w233 w236] -> w200
                  frame #0 {
                    n76 = call-poly <vilib>:"Convolution.vi"("Y"=w212, "X"=w213) -> ("X * Y"=w210:dbl[])  [unwired: 8 in, 1 out]
                  }
                  frame #1 {
                    n77 = Compound Arithmetic op=ADD(w217, w216) -> (w214:dbl[])
                  }
                  frame #2 {
                    n78 = Compound Arithmetic op=MULTIPLY(w221, w220) -> (w218:dbl[])
                  }
                  frame #3 {
                    n79 = call "backward difference system.vi"("Input sequence x[n]"=w225) -> ("B[n] = x[n] - x[n-1]"=w222:dbl[])
                  }
                  frame #4 {
                    n80 = call "accumulator system.vi"("Sequence x[n]"=w229) -> ("Accumulated sequence A[n] = Sum(k: k ( -infinity to n) x[k]"=w226:dbl[])  [unwired: 2 out]
                  }
                  frame #5 {
                    n81 = call-poly <vilib>:"CrossCorrelation.vi"("Y"=w231, "X"=w232) -> ("Rxy"=w233:dbl[])  [unwired: 8 in, 1 out]
                  }
                  frame #6 {
                    n82 = call-poly <vilib>:"AutoCorrelation.vi"("X"=w237) -> ("Rxx"=w236:dbl[])  [unwired: 9 in, 1 out]
                  }
                }
                n83 = call "Convert to Dynamic Data6"("Array"=w203) -> ("Dynamic Data Type"=w206:dynamicdata)  [unwired: 3 in]
                n84 = call "Convert to Dynamic Data7"("Array"=w204) -> ("Dynamic Data Type"=w205:dynamicdata)  [unwired: 3 in]
                n85 = Merge Signals(w206, w205) -> (w202:dynamicdata)
              }
              frame #3 {
                n86 = case shown="\"MULTIPLICATION\"" w247 {
                  tunnel: w249 -> [w253 w257 w261 w265 w269 w271 w277]
                  tunnel: w248 -> [w252 w256 w260 _ _ w270 _]
                  tunnel: [w250 w254 w258 w262 w266 w273 w275] -> w246
                  tunnel: [w253 w257 w261 w265 w269 w271 w277] -> w244
                  tunnel: [w252 w256 w260 dbl[] [0.0, 0.0, 0.0, 0.0, 0.0, 0.0, 0.0, 0.0, 0.0, 0.0, 0.0, 0.0, 0.0, 0.0, 0.0, 0.0, 0.0, 0.0, 0.0, 0.0, 0.0, 0.0, 0.0, 0.0, 0.0, 0.0, 0.0, 0.0, 0.0, 0.0, 0.0, 0.0, 0.0, 0.0, 0.0, 0.0, 0.0, 0.0, 0.0, 0.0, 0.0, 0.0, 0.0, 0.0, 0.0, 0.0, 0.0, 0.0, 0.0, 0.0, 0.0, 0.0, 0.0, 0.0, 0.0, 0.0, 0.0, 0.0, 0.0, 0.0, 0.0, 0.0, 0.0, 0.0, 0.0, 0.0, 0.0, 0.0, 0.0, 0.0, 0.0, 0.0, 0.0, 0.0, 0.0, 0.0, 0.0, 0.0, 0.0, 0.0, 0.0, 0.0, 0.0, 0.0, 0.0, 0.0, 0.0, 0.0, 0.0, 0.0, 0.0, 0.0, 0.0, 0.0, 0.0, 0.0, 0.0, 0.0, 0.0, 0.0, 0.0] dbl[] [0.0, 0.0, 0.0, 0.0, 0.0, 0.0, 0.0, 0.0, 0.0, 0.0, 0.0, 0.0, 0.0, 0.0, 0.0, 0.0, 0.0, 0.0, 0.0, 0.0, 0.0, 0.0, 0.0, 0.0, 0.0, 0.0, 0.0, 0.0, 0.0, 0.0, 0.0, 0.0, 0.0, 0.0, 0.0, 0.0, 0.0, 0.0, 0.0, 0.0, 0.0, 0.0, 0.0, 0.0, 0.0, 0.0, 0.0, 0.0, 0.0, 0.0, 0.0, 0.0, 0.0, 0.0, 0.0, 0.0, 0.0, 0.0, 0.0, 0.0, 0.0, 0.0, 0.0, 0.0, 0.0, 0.0, 0.0, 0.0, 0.0, 0.0, 0.0, 0.0, 0.0, 0.0, 0.0, 0.0, 0.0, 0.0, 0.0, 0.0, 0.0, 0.0, 0.0, 0.0, 0.0, 0.0, 0.0, 0.0, 0.0, 0.0, 0.0, 0.0, 0.0, 0.0, 0.0, 0.0, 0.0, 0.0, 0.0, 0.0, 0.0] w270 dbl[] [0.0, 0.0, 0.0, 0.0, 0.0, 0.0, 0.0, 0.0, 0.0, 0.0, 0.0, 0.0, 0.0, 0.0, 0.0, 0.0, 0.0, 0.0, 0.0, 0.0, 0.0, 0.0, 0.0, 0.0, 0.0, 0.0, 0.0, 0.0, 0.0, 0.0, 0.0, 0.0, 0.0, 0.0, 0.0, 0.0, 0.0, 0.0, 0.0, 0.0, 0.0, 0.0, 0.0, 0.0, 0.0, 0.0, 0.0, 0.0, 0.0, 0.0, 0.0, 0.0, 0.0, 0.0, 0.0, 0.0, 0.0, 0.0, 0.0, 0.0, 0.0, 0.0, 0.0, 0.0, 0.0, 0.0, 0.0, 0.0, 0.0, 0.0, 0.0, 0.0, 0.0, 0.0, 0.0, 0.0, 0.0, 0.0, 0.0, 0.0, 0.0, 0.0, 0.0, 0.0, 0.0, 0.0, 0.0, 0.0, 0.0, 0.0, 0.0, 0.0, 0.0, 0.0, 0.0, 0.0, 0.0, 0.0, 0.0, 0.0, 0.0]] -> w242
                  tunnel: ["CONVOLUTION    " "ADDITION       " "MULTIPLICATION    " "BACKWARD DIFFERENCE    " "ACCUMULATOR\n     " "CROSS CORRELATION" "AUTO CORRELATION"] -> w239
                  tunnel: [w250 w254 w258 w262 w266 w273 w275] -> w238
                  frame #0 {
                    n87 = call-poly <vilib>:"Convolution.vi"("Y"=w252, "X"=w253) -> ("X * Y"=w250:dbl[])  [unwired: 8 in, 1 out]
                  }
                  frame #1 {
                    n88 = Compound Arithmetic op=ADD(w257, w256) -> (w254:dbl[])
                  }
                  frame #2 {
                    n89 = Compound Arithmetic op=MULTIPLY(w261, w260) -> (w258:dbl[])
                  }
                  frame #3 {
                    n90 = call "backward difference system.vi"("Input sequence x[n]"=w265) -> ("B[n] = x[n] - x[n-1]"=w262:dbl[])
                  }
                  frame #4 {
                    n91 = call "accumulator system.vi"("Sequence x[n]"=w269) -> ("Accumulated sequence A[n] = Sum(k: k ( -infinity to n) x[k]"=w266:dbl[])  [unwired: 2 out]
                  }
                  frame #5 {
                    n92 = call-poly <vilib>:"CrossCorrelation.vi"("Y"=w270, "X"=w271) -> ("Rxy"=w273:dbl[])  [unwired: 8 in, 1 out]
                  }
                  frame #6 {
                    n93 = call-poly <vilib>:"AutoCorrelation.vi"("X"=w277) -> ("Rxx"=w275:dbl[])  [unwired: 9 in, 1 out]
                  }
                }
                n94 = call "Convert to Dynamic Data"("Array"=w246) -> ("Dynamic Data Type"=w245:dynamicdata)  [unwired: 3 in]
                n95 = call "Convert to Dynamic Data3"("Array"=w242) -> ("Dynamic Data Type"=w241:dynamicdata)  [unwired: 3 in]
                n96 = call "Convert to Dynamic Data2"("Array"=w244) -> ("Dynamic Data Type"=w243:dynamicdata)  [unwired: 3 in]
                n97 = Merge Signals(w243, w245, w241) -> (w240:dynamicdata)
              }
            }
          }
        }
      }
    }
    "OUTPUT ARRAY" <- w34
    n98 = Reciprocal(x="Samp freq Fs") -> (1/x=w12:dbl)
    n99 = Reciprocal(x="Samp freq Fs") -> (1/x=w22:dbl)
    n100 = case shown="True" "?" {
      tunnel: w33 -> [w89 w90]
      tunnel: [w86 w90] -> w16
      frame #0 {
        n101 = Logarithm Base 10(1:w89) -> (0:w88:dynamicdata)
        n102 = Multiply(x=w88, y=20) -> (x*y=w86:dynamicdata)
      }
      frame #1 {
      }
    }
    "Signal Operation (x,y)" <- w16
    n103 = case shown="False" w5 {
      tunnel: [w51 w53] -> w3
      tunnel: w4 -> [w51 _]
      tunnel: [FALSE TRUE] -> w2
      frame #0 {
      }
      frame #1 {
        w53 = "Warning: Analog Freq > (Samp Freq/2)\nAliasing my occur at the Input."  # Warning: Analog Freq > (Samp Freq/2) Aliasing my occur at the Input.
      }
    }
    "?" <- w2
    "?" <- w3
    n104 = case shown="True" "?" {
      tunnel: w36 -> [w68 w73]
      tunnel: w22 -> [w67 _]
      tunnel: [w65 w70] -> w21
      tunnel: ["Time" "Samples"] -> w19
      frame #0 {
        n105 = Bundle(0.0, w67, "Chirp Pattern"=w68) -> (w65:cluster{dbl, dbl, "Chirp Pattern":dbl[]})  [unwired: 1 in]
      }
      frame #1 {
        n106 = Bundle(0.0, 1.0, "Chirp Pattern"=w73) -> (w70:cluster{dbl, dbl, "Chirp Pattern":dbl[]})  [unwired: 1 in]
      }
    }
    "Sequence x[n]" <- w21
    "?" <- w19
    n107 = case shown="True" "?" {
      tunnel: [w54 w61] -> w14
      tunnel: ["Time" "Samples"] -> w18
      tunnel: w15 -> [w56 w59]
      tunnel: w12 -> [w55 _]
      frame #0 {
        n108 = Bundle(0.0, w55, "poisson noise"=w56) -> (w54:cluster{dbl, dbl, "poisson noise":dbl[]})  [unwired: 1 in]
      }
      frame #1 {
        n109 = Bundle(0.0, 1.0, "poisson noise"=w59) -> (w61:cluster{dbl, dbl, "poisson noise":dbl[]})  [unwired: 1 in]
      }
    }
    "?" <- w18
    "Sequence y[n]" <- w14
  }
